vi "Execute Value Update Policy.vi"(8 "error in (no error)":errorcluster, 9 "Publish Time":timestamp, 10 "New Topic Value":variant, 11 "TriggeredSubscription In":refnum<class "TriggeredSubscription.lvclass">) -> (0 "error out":errorcluster, 3 "TriggeredSubscription Out":refnum<class "TriggeredSubscription.lvclass">)   [LabVIEW 2018, in "MVA Framework.lvlib" / "SubscriptionPolicy.lvlib" / "TriggeredSubscription.lvclass"]
doc: "执行值更新策略"
uses:
  TriggeredSubscription.lvclass
  IMediator/ISubscriptionPolicy/ISubscriptionPolicy.lvclass
  <vilib>/ErrorRing/Error Ring.xnode
  <vilib>/Utility/error.llb/Error Cluster From Error Code.vi
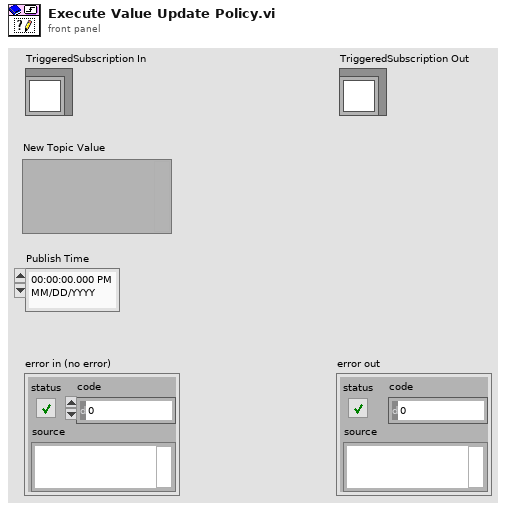
[diagram p1: front panel]
types:
  T1 = enum16{"Equal", "Not equal", "Greater than", "Less than", "Greater or equal", "Less or equal"}
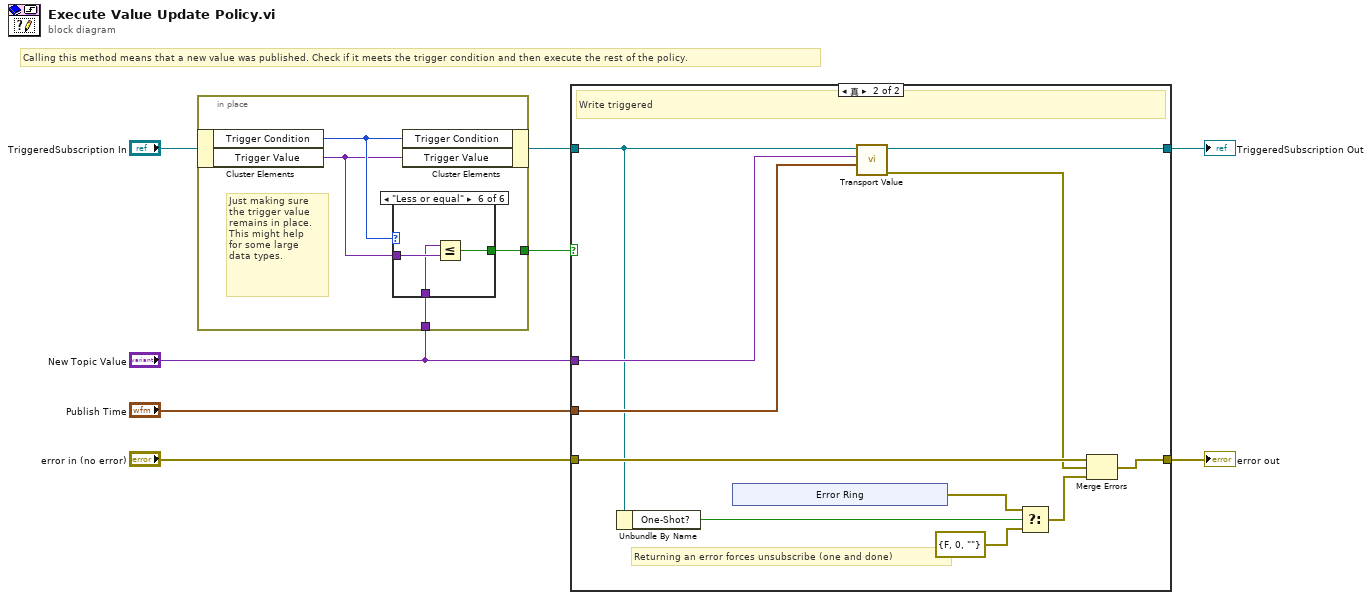
[diagram p0: block diagram]
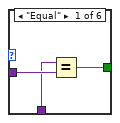
[diagram p2: hidden frame]
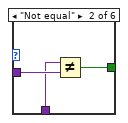
[diagram p3: hidden frame]
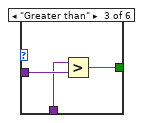
[diagram p4: hidden frame]
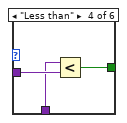
[diagram p5: hidden frame]
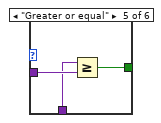
[diagram p6: hidden frame]
diagram:
  # "Calling this method means that a new value was published. Check if it meets the trigger condition and then execute the rest of the policy."
  n1 = in-place {
    in-place-border: "New Topic Value" -> [w12]
    in-place-border: [w11] -> w3
    # "Just making sure\nthe trigger value\nremains in place.\nThis might help\nfor some large\ndata types."
    n2 = in-place-cluster #1("TriggeredSubscription In") -> ("Trigger Condition"=w10:T1, "Trigger Value"=w9:variant)
    n3 = case shown="\"Less or equal\"" w10 {
      tunnel: w9 -> [w15 w18 w21 w24 w27 w30]
      tunnel: w12 -> [w14 w17 w20 w23 w26 w29]
      tunnel: [w13 w16 w19 w22 w25 w28] -> w11
      frame "Equal" {
        n4 = Equal?(x=w14, y=w15) -> (x = y?=w13:bool)
      }
      frame "Not equal" {
        n5 = Not Equal?(x=w17, y=w18) -> (x != y?=w16:bool)
      }
      frame "Greater than" {
        n6 = Greater?(x=w20, y=w21) -> (0:w19:bool)
      }
      frame "Less than" {
        n7 = Less?(x=w23, y=w24) -> (x < y?=w22:bool)
      }
      frame "Greater or equal" {
        n8 = Greater Or Equal?(x=w26, y=w27) -> (x >= y?=w25:bool)
      }
      frame "Less or equal" {
        n9 = Less Or Equal?(x=w29, y=w30) -> (x <= y?=w28:bool)
      }
    }
    n10 = in-place-cluster #1("Trigger Condition"=w10, "Trigger Value"=w9) -> (w1:refnum<class "TriggeredSubscription.lvclass">)
  }
  n11 = case shown="真" w3 {
    tunnel: "Publish Time" -> [_ w35]
    tunnel: "error in (no error)" -> [w32 w43]
    tunnel: [w32 w42] -> w6
    tunnel: "New Topic Value" -> [_ w36]
    tunnel: [w31 w37] -> w4
    tunnel: w1 -> [w31 w33]
    frame False {
      # "Write NOT triggered"
    }
    frame True {
      # "Returning an error forces unsubscribe (one and done)"
      # "Write triggered"
      n12 = Unbundle By Name(w33) -> ("One-Shot?"=w41:bool)
      n13 = xnode "Error Ring"() -> ("错误输出"=w39:errorcluster)
      n14 = call "Transport Value.vi"("Publish Time"=w35, "Value"=w36, "ISubscriptionPolicy in"=w33) -> ("error out"=w34:errorcluster, "ISubscriptionPolicy out"=w37:refnum<class "TriggeredSubscription.lvclass">)  [unwired: 7 in]
      n15 = Select(t=w39, s=w41, f=errorcluster {"status"=FALSE, "code"=0, "source"=""}) -> (s? t:f=w40:errorcluster)
      n16 = Merge Errors(w43, w34, w40) -> (w42:errorcluster)
    }
  }
  "error out" <- w6
  "TriggeredSubscription Out" <- w4
